vi "Rotate2Darray.vi"(0 "Color Table Index of Fill Color":i32, 1 "Angle":dbl=3.141592 format="%.6f", 2 "Array In":i32[][](array[numeric])=[[11, 12, 13, 14], [21, 22, 23, 24], [31, 32, 33, 34], [41, 42, 43, 44]], 3 "Maintain Center Position?":bool=TRUE) -> (4 "Array Out":u32[][](array[numeric])=[[0, 0], [0, 4]])   [LabVIEW 2011]
doc: "Component of \"Rotate Pixmap.VI\". Used for 24 bit pixmaps."
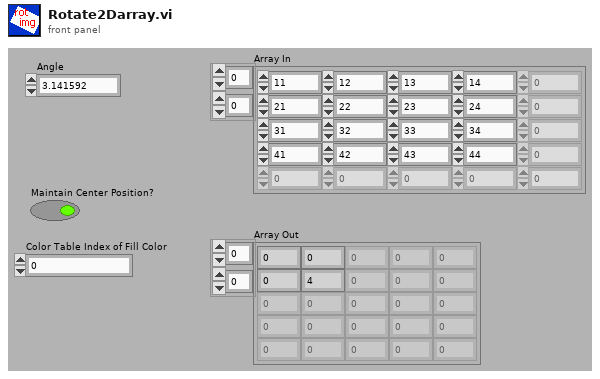
[diagram p1: front panel]
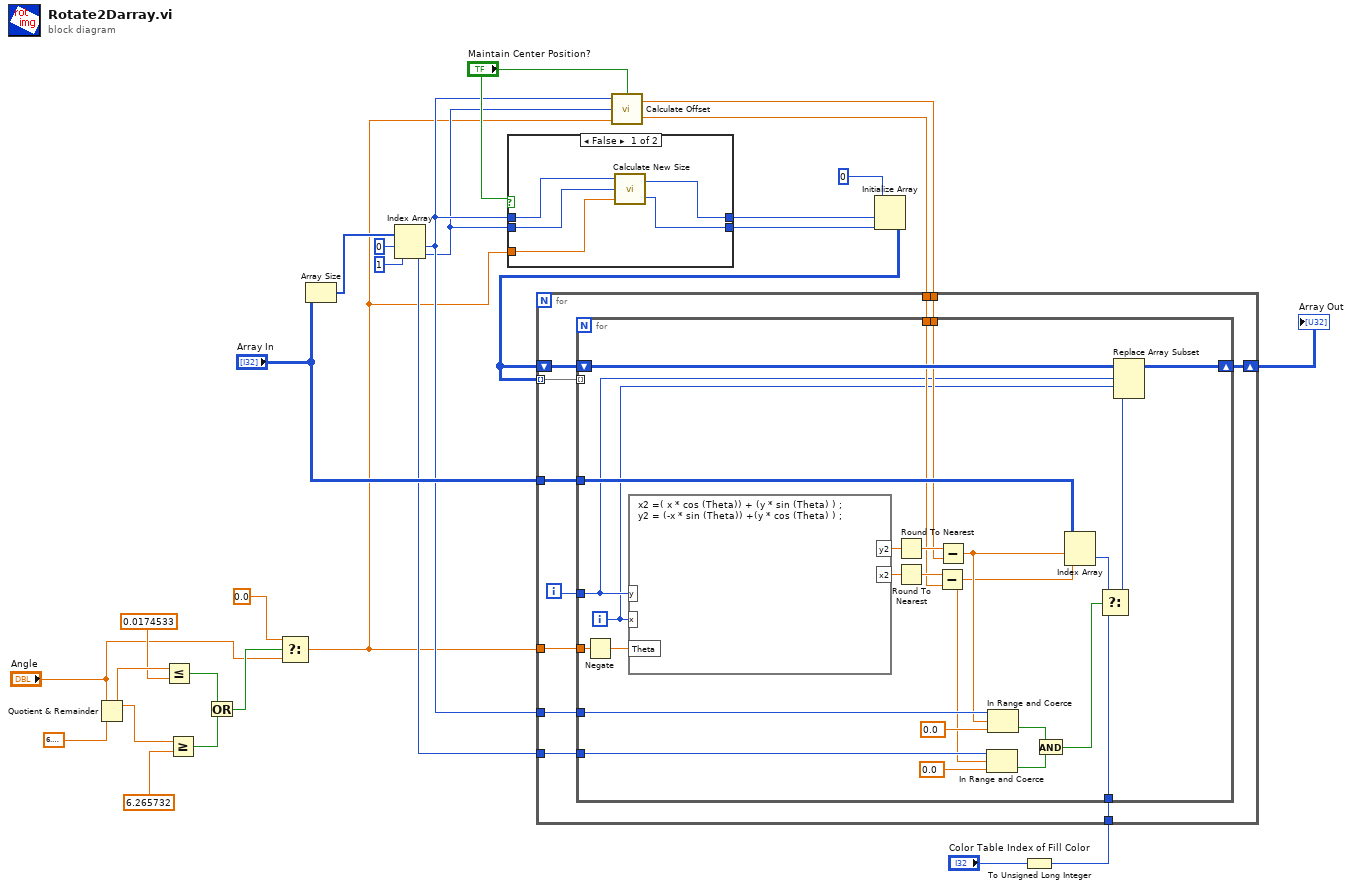
[diagram p0: block diagram]
diagram:
  n1 = Quotient & Remainder(x="Angle", y=6.283185307179586) -> (x-y*floor(x/y)=w9:dbl)  [unwired: 1 out]
  n2 = Less Or Equal?(x=w9, y=0.0174533) -> (x <= y?=w8:bool)
  n3 = Greater Or Equal?(x=w9, y=6.265732) -> (x >= y?=w7:bool)
  n4 = Or(x=w8, y=w7) -> (x .or. y?=w4:bool)
  n5 = Select(t=0.0, s=w4, f="Angle") -> (s? t:f=w1:dbl)
  n6 = Array Size(array="Array In") -> (size(s)=w21:i32[])
  n7 = Index Array(array=w21, index #1=0 ("Index"), index #2=1 ("Index")) -> (element #1=w13:i32, element #2=w12:i32)
  n8 = case shown="False" "Maintain Center Position?" {
    tunnel: w13 -> [w30 w33]
    tunnel: w12 -> [w29 w32]
    tunnel: [w28 w33] -> w18
    tunnel: [w27 w32] -> w17
    tunnel: w1 -> [w31 _]
    frame False {
      n9 = call "Calculate New Size.vi"("Angle (radians)"=w31, "Width"=w29, "Heigt"=w30) -> ("New Width"=w27:i32, "New Height"=w28:i32)
    }
    frame True {
    }
  }
  n10 = call "Calculate Offset.vi"("Maintain Center Position?"="Maintain Center Position?", "Angle (radians)"=w1, "Width"=w12, "Hight"=w13) -> ("Offset x"=w15:dbl, "Offset y"=w14:dbl)
  n11 = Initialize Array(u32 0, w18, w17) -> (w16:u32[][])
  n12 = To Unsigned Long Integer(number="Color Table Index of Fill Color") -> (unsigned 32bit integer=w22:u32)
  n13 = for {
    tunnel: "Array In" -> [w44]
    tunnel: w1 -> [w39]
    shift-right: [w42] -> w11
    shift-left: w16 -> [w41]
    tunnel: w16 -> [w40] mode=indexing
    tunnel: w14 -> [w38]
    tunnel: w15 -> [w37]
    tunnel: w12 -> [w36]
    tunnel: w13 -> [w35]
    tunnel: w22 -> [w34]
    i -> [w43]
    n14 = for {
      tunnel: w44 -> [w65]
      tunnel: w43 -> [w48]
      tunnel: w39 -> [w46]
      shift-right: [w67] -> w42
      shift-left: w41 -> [w66]
      tunnel: w40 -> [_] mode=indexing
      tunnel: w38 -> [w62]
      tunnel: w37 -> [w61]
      tunnel: w36 -> [w58]
      tunnel: w35 -> [w59]
      tunnel: w34 -> [w51]
      i -> [w47]
      n15 = Negate(x=w46) -> (-x=w45:dbl)
      n16 = formula code="x2 =( x * cos (Theta)) + (y * sin (Theta) ) ;\ny2 = (-x * sin (Theta)) +(y * cos (Theta) ) ;"("y"=w48, "x"=w47, "Theta"=w45) -> ("y2"=w69:dbl, "x2"=w68:dbl)
      n17 = Round To Nearest(number=w69) -> (nearest integer value=w64:dbl)
      n18 = Round To Nearest(number=w68) -> (nearest integer value=w63:dbl)
      n19 = Subtract(x=w63, y=w61) -> (x-y=w49:dbl)
      n20 = Subtract(x=w64, y=w62) -> (x-y=w50:dbl)
      n21 = In Range and Coerce(upper limit=w58, x=w49, lower limit=0.0) -> (In Range?=w54:bool)  [unwired: 1 out]
      n22 = In Range and Coerce(upper limit=w59, x=w50, lower limit=0.0) -> (In Range?=w55:bool)  [unwired: 1 out]
      n23 = And(x=w55, y=w54) -> (x .and. y?=w53:bool)
      n24 = Index Array(array=w65, index (row)=w50, index (col)=w49) -> (element=w56:i32)
      n25 = Select(t=w56, s=w53, f=w51) -> (s? t:f=w52:u32)
      n26 = Replace Array Subset(array=w66, new element=w52, index (row)=w48, index (col)=w47) -> (w67:u32[][])
    }
  }
  "Array Out" <- w11
